vi "ScaleNoiseParams.vi"(0 "WhiteNoise":cluster{"Vpeak (V)":u16, "Seed":u32}={"Vpeak (V)"=5, "Seed"=10}, 5 "max voltage for target":dbl=10.0, 11 "error in (no error)":errorcluster) -> (4 "scaled square wave props":cluster{"amplitude":u16, "seed":u32}, 15 "error out":errorcluster)   [LabVIEW 2021]
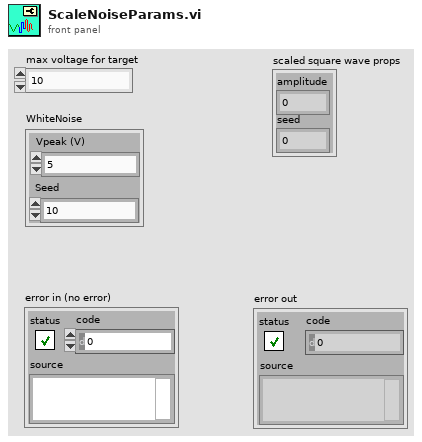
[diagram p1: front panel]
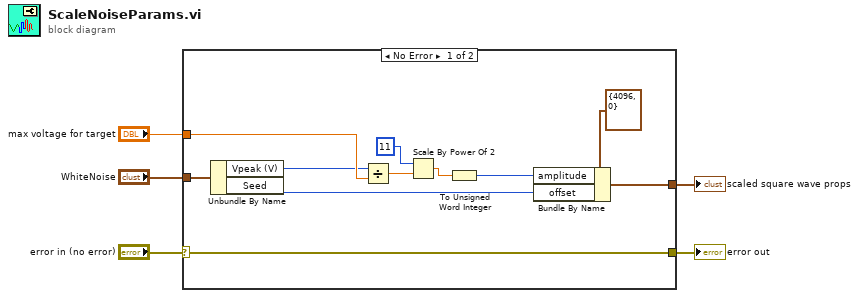
[diagram p0: block diagram]
diagram:
  n1 = case shown="No Error" "error in (no error)" {
    selector: "error in (no error)" -> [w7 w17]
    tunnel: [w16 _] -> w5
    tunnel: "WhiteNoise" -> [w12 _]
    tunnel: "max voltage for target" -> [w11 _]
    tunnel: [w7 w17] -> w2
    frame No Error {
      n2 = Unbundle By Name(w12) -> ("Vpeak (V)"=w6:u16, "Seed"=w8:u32)
      n3 = Divide(x=w6, y=w11) -> (x/y=w15:dbl)
      n4 = Scale By Power Of 2(n=11, x=w15) -> (x*2^n=w13:dbl)
      n5 = To Unsigned Word Integer(number=w13) -> (unsigned 16bit integer=w9:u16)
      n6 = Bundle By Name(cluster=cluster{"amplitude":u16, "offset":u32} {"amplitude"=4096, "offset"=0} ("Square wave 3"), "amplitude"=w9, "offset"=w8) -> (w16:cluster{"amplitude":u16, "offset":u32})
    }
    frame Error {
    }
  }
  "scaled square wave props" <- w5
  "error out" <- w2
